vi "Open.vi"(5 "Output Data Rate (Hz)":enum16{"400", "200", "100", "50", "25", "12.5"}(ring)=enum."100", 7 "SPI Channel (0)":u8, 8 "Error In (no error)":errorcluster, 9 "Resolution (g)":enum16{"8g", "4g", "2g"}(ring)=enum."2g", 10 "CS Channel":u8, 11 "LINX Resource":T1) -> (0 "Error Out":errorcluster, 1 "Resolution (g)":enum16{"8g", "4g", "2g"}(ring), 3 "LINX Resource":T1)   [LabVIEW 2020, in "LMH-LINX.lvlib" / "PmodACL2.lvlib"]
doc: "Opens the PmodACL2 with correct settings.\nSCL = 1MHz to 8MHz (set to 1MHz)\nLSb FIrst\nMode 0\nActive Low\n\nUser selects output data rate and resolution and writes to register 0x2C using the write command 0xA\nWrites 0x2 to register 0x2D to tell the PmodACL2 to enter measurement mode"
uses:
  PmodACL2.lvlib
  Private/Type Defs/LINX Ref.ctl
  Private/Type Defs/Platform.ctl
  Private/Type Defs/Interface.ctl
  Private/Device/Type Defs/LINX Device Config.ctl
  Private/Device/Type Defs/TCP Config.ctl
  Private/Device/Type Defs/Channels.ctl
  Peripherals/SPI/SPI CS Config.ctl
  Private/Type Defs/Peripherals/SPI/SPI CS Logic Level.ctl
  Private/Type Defs/Peripherals/SPI/SPI Configuration.ctl
  Private/Type Defs/Peripherals/SPI/SPI Bit Order.ctl
  Private/Type Defs/Peripherals/SPI/SPI Mode.ctl
  Peripherals/SPI/SPI Write Read 1 Frame.vi
  Peripherals/SPI/SPI Write Read N Frames.vi
  Private/Local IO/LinxSpiWriteRead.vi
  Utilities/Check Channel.vi
  Private/Utilties/Generate Error.vi
  LMH-LINX.lvlib
  Private/Device/Device.lvlib
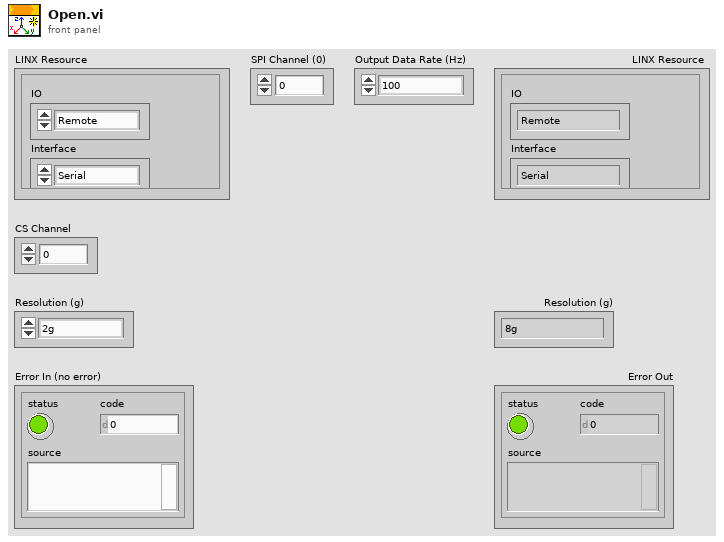
[diagram p1: front panel]
types:
  T1 = typedef "LMH-LINX.lvlib/LINX Ref.ctl" = cluster{"IO":T2, "Interface":T3, "LINX Device Config":T4}
  T2 = typedef "LMH-LINX.lvlib/Platform.ctl" = enum16{"Remote", "Local"}
  T3 = typedef "LMH-LINX.lvlib/Interface.ctl" = enum16{"Serial", "TCP"}
  T4 = typedef "Device.lvlib/LINX Device Config.ctl" = cluster{"Interface":T3, "COM Port":refnum<visa-resource-name>, "TCP Configuration":T5, "Device Family":u8, "Device ID":u8, "Device Name":string, "TCP Ref":refnum<k5>, "Channels":T6}
  T5 = typedef "Device.lvlib/TCP Config.ctl" = cluster{"IP Address":string, "Port":u16}
  T6 = typedef "LMH-LINX.lvlib/Channels.ctl" = cluster{"DI":u8[], "DO":u8[], "AI":u8[], "AO":u8[], "PWM":u8[], "QE":u8[], "UART":u8[], "I2C 2":u8[], "SPI":u8[], "CAN":u8[], "Servo":u8[], "AI Ref (V)":dbl, "AI Resolution (Bits)":u8, "AO Ref (V)":dbl, "AO Resolution (Bits)":u8}
  T7 = typedef "LMH-LINX.lvlib/SPI Configuration.ctl" = cluster{"Clock Frequency":u32, "Bit Order":T8, "SPI Mode":T9}
  T8 = typedef "LMH-LINX.lvlib/SPI Bit Order.ctl" = enum8{"LSb First", "MSb First"}
  T9 = typedef "LMH-LINX.lvlib/SPI Mode.ctl" = enum8{"Mode 0", "Mode 1", "Mode 2", "Mode 3"}
  T10 = typedef "LMH-LINX.lvlib/SPI CS Config.ctl" = cluster{"CS Channel":u8, "CS Logic Level":T11}
  T11 = typedef "LMH-LINX.lvlib/SPI CS Logic Level.ctl" = enum8{"Active Low", "Active High"}
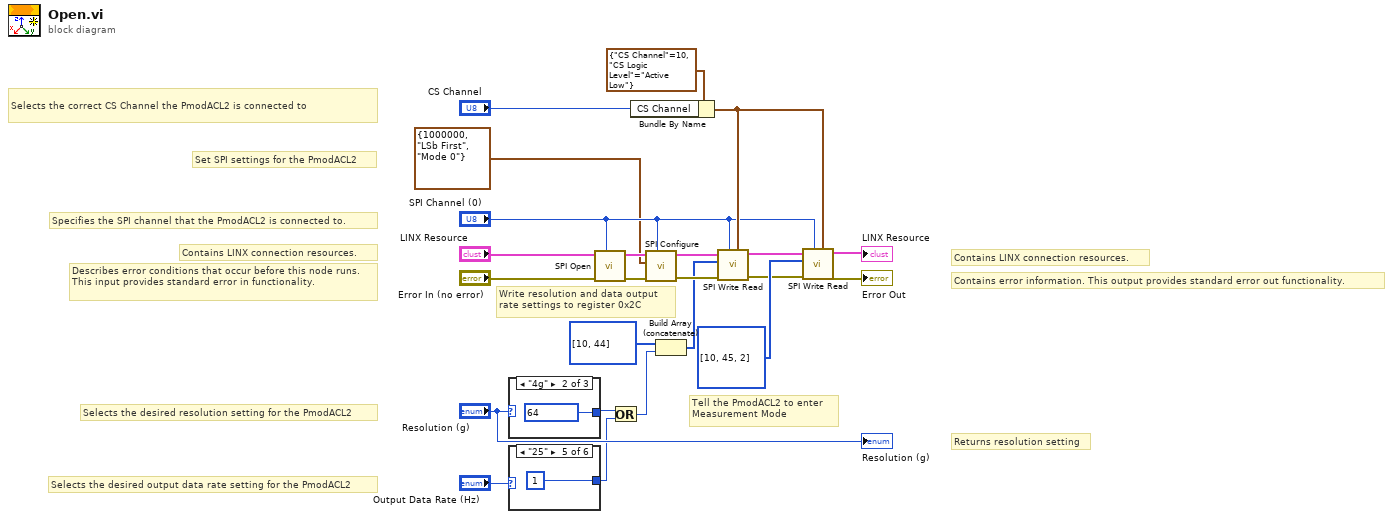
[diagram p0: block diagram]
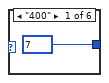
[diagram p2: hidden frame]
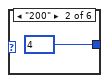
[diagram p3: hidden frame]
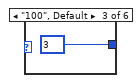
[diagram p4: hidden frame]
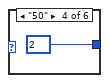
[diagram p5: hidden frame]
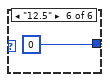
[diagram p6: hidden frame]
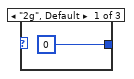
[diagram p7: hidden frame]
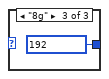
[diagram p8: hidden frame]
diagram:
  # "Tell the PmodACL2 to enter\nMeasurement Mode"
  # "Write resolution and data output \nrate settings to register 0x2C"
  # "Selects the desired output data rate setting for the PmodACL2"
  # "Selects the desired resolution setting for the PmodACL2"
  # "Returns resolution setting"
  # "Contains LINX connection resources."
  # "Contains error information. This output provides standard error out functionality."
  # "Selects the correct CS Channel the PmodACL2 is connected to"
  # "Set SPI settings for the PmodACL2"
  # "Specifies the SPI channel that the PmodACL2 is connected to."
  # "Contains LINX connection resources."
  # "Describes error conditions that occur before this node runs. This input provides standard error in functionality."
  n1 = case shown="\"4g\"" "Resolution (g)" {
    tunnel: [u8 0 u8 64 u8 192] -> w4
    frame "2g", Default {
    }
    frame "4g" {
    }
    frame "8g" {
    }
  }
  n2 = case shown="\"25\"" "Output Data Rate (Hz)" {
    tunnel: [u8 7 u8 4 u8 3 u8 2 u8 1 u8 0] -> w3
    frame "400" {
    }
    frame "200" {
    }
    frame "100", Default {
    }
    frame "50" {
    }
    frame "25" {
    }
    frame "12.5" {
    }
  }
  n3 = call "SPI Open.vi"("SPI Channel (0)"="SPI Channel (0)", "Error In"="Error In (no error)", "LINX Resource"="LINX Resource") -> ("Error Out"=w7:errorcluster, "LINX Resource"=w6:T1)  [unwired: 7 in]
  n4 = Or(x=w4, y=w3) -> (x .or. y?=w2:u8)
  n5 = Bundle By Name(cluster=T10 {"CS Channel"=10, "CS Logic Level"=enum."Active Low"} ("CS Configuration"), "CS Channel"="CS Channel") -> (w23:T10)
  n6 = call "SPI Configure.vi"("SPI Channel (0)"="SPI Channel (0)", "Error In"=w7, "SPI Configuration"=T7 {"Clock Frequency"=1000000, "Bit Order"=enum."LSb First", "SPI Mode"=enum."Mode 0"}, "LINX Resource"=w6) -> ("Error Out"=w11:errorcluster, "LINX Resource"=w10:T1)  [unwired: 5 in, 1 out]
  n7 = Build Array (concatenate)(u8[] [10, 44] ("Data"), w2) -> (w1:u8[])
  n8 = call-poly "SPI Write Read.vi"("CS Configuration"=w23, "SPI Channel (0)"="SPI Channel (0)", "Error In"=w11, "Data"=w1, "LINX Resource"=w10) -> ("Error Out"=w14:errorcluster, "LINX Resource"=w13:T1)  [unwired: 3 in, 2 out]
  n9 = call-poly "SPI Write Read.vi"("CS Configuration"=w23, "SPI Channel (0)"="SPI Channel (0)", "Error In"=w14, "Data"=u8[] [10, 45, 2], "LINX Resource"=w13) -> ("Error Out"=→"Error Out":errorcluster, "LINX Resource"=→"LINX Resource":T1)  [unwired: 3 in, 2 out]
  "Resolution (g)" <- "Resolution (g)"
